vi "Sub_time_correction_2022.vi"(2 "Experimental Results IN":T1={"time_average_cycle"=0.0, "measured_frequency"=[], "date_time"="", "estimated_pin_node"=[], "time_cycle_start"=[], "measured_pin_location"=[], "estimated_frequency"=[], "acceleration_data"=[], "accelerometer_sample_rate"=0.0, "displacement_sample_rate"=0.0, "time_compare_start"=array[564 elements], "time_subsample_start"=array[564 elements], "time_FEA_start"=array[564 elements], "time_FEA_end"=array[564 elements], "time_cycle_end"=array[564 elements], "time_accelerometer_aquire_start"=array[564 elements], "time_frequency_calculations_start"=array[564 elements], "time_frequency_calculations_end"=array[564 elements], "measured_pin_location_tt"=array[564 elements], "time_ACC_data_collection_start"=0.0, "time_acceleration_data"=array[564 elements], "estimated_pin_location"=array[564 elements], "scaling_factor_Hz_per_pin_to_frequency_resolution"=1.0, "Std_Dev_equale_particles_divided_3"=TRUE, "Auto_FFT_length"=TRUE, "windowed_acc_data"=array1x564[564 elements], "FFT"=array1x564[564 elements]}) -> (16 "Experimental Results OUT":T1={"time_average_cycle"=0.0, "measured_frequency"=[], "date_time"="", "estimated_pin_node"=[], "time_cycle_start"=[], "measured_pin_location"=[], "estimated_frequency"=[], "acceleration_data"=[], "accelerometer_sample_rate"=0.0, "displacement_sample_rate"=0.0, "time_compare_start"=array[564 elements], "time_subsample_start"=array[564 elements], "time_FEA_start"=array[564 elements], "time_FEA_end"=array[564 elements], "time_cycle_end"=array[564 elements], "time_accelerometer_aquire_start"=array[564 elements], "time_frequency_calculations_start"=array[564 elements], "time_frequency_calculations_end"=array[564 elements], "measured_pin_location_tt"=array[564 elements], "time_ACC_data_collection_start"=0.0, "time_acceleration_data"=array[564 elements], "estimated_pin_location"=array[564 elements], "scaling_factor_Hz_per_pin_to_frequency_resolution"=1.0, "Std_Dev_equale_particles_divided_3"=TRUE, "Auto_FFT_length"=TRUE, "windowed_acc_data"=array1x564[564 elements], "FFT"=array1x564[564 elements]})   [LabVIEW 2019]
uses:
  <vilib>/Analysis/baseanly.llb/Mean (DBL).vi
  <vilib>/Analysis/NI_AALBase.lvlib
panel:
  out "mean":dbl format="%0.10f"
  out "number of iterations run":i32
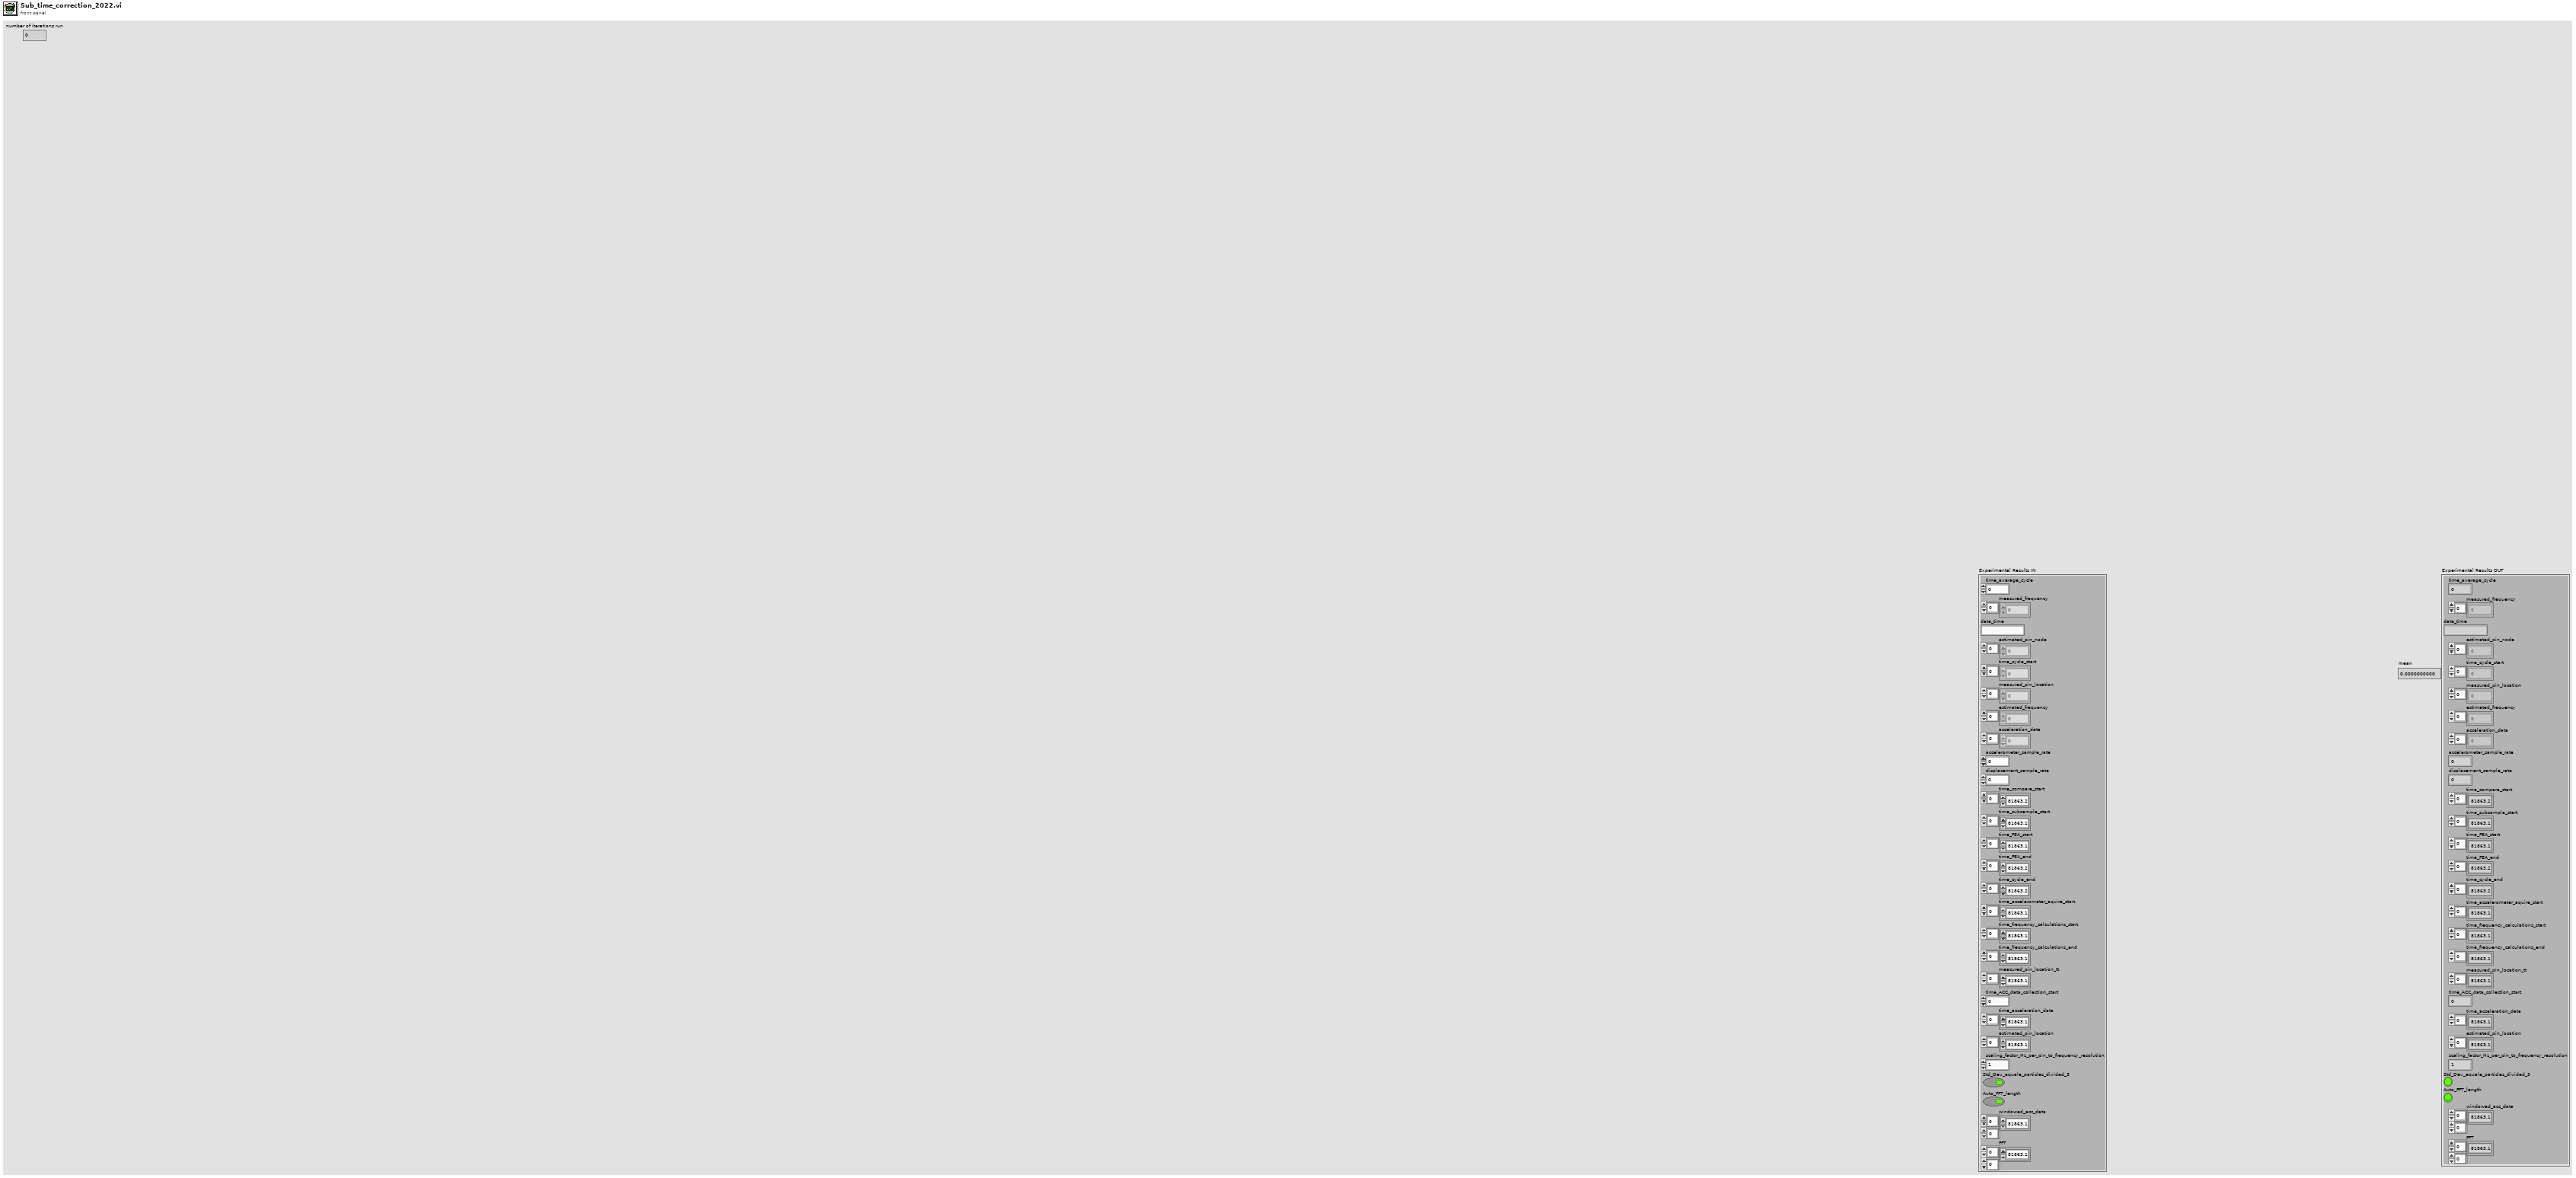
[diagram p1: front panel]
types:
  T1 = cluster{"time_average_cycle":dbl, "measured_frequency":dbl[], "date_time":string, "estimated_pin_node":i32[], "time_cycle_start":dbl[], "measured_pin_location":dbl[], "estimated_frequency":dbl[], "acceleration_data":dbl[], "accelerometer_sample_rate":dbl, "displacement_sample_rate":dbl, "time_compare_start":dbl[], "time_subsample_start":dbl[], "time_FEA_start":dbl[], "time_FEA_end":dbl[], "time_cycle_end":dbl[], "time_accelerometer_aquire_start":dbl[], "time_frequency_calculations_start":dbl[], "time_frequency_calculations_end":dbl[], "measured_pin_location_tt":dbl[], "time_ACC_data_collection_start":dbl, "time_acceleration_data":dbl[], "estimated_pin_location":dbl[], "scaling_factor_Hz_per_pin_to_frequency_resolution":dbl, "Std_Dev_equale_particles_divided_3":bool, "Auto_FFT_length":bool, "windowed_acc_data":dbl[][], "FFT":dbl[][]}
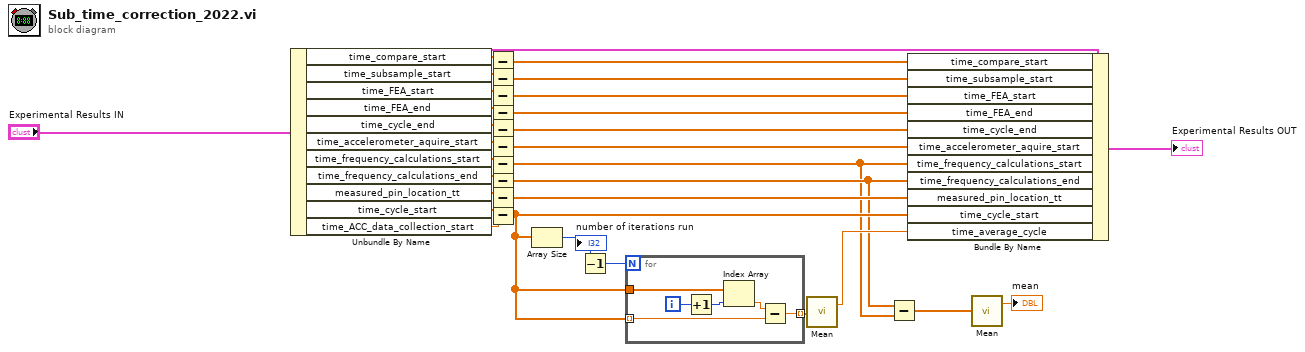
[diagram p0: block diagram]
diagram:
  n1 = Unbundle By Name("Experimental Results IN") -> ("time_compare_start"=w2:dbl[], "time_subsample_start"=w3:dbl[], "time_FEA_start"=w4:dbl[], "time_FEA_end"=w5:dbl[], "time_cycle_end"=w6:dbl[], "time_accelerometer_aquire_start"=w7:dbl[], "time_frequency_calculations_start"=w8:dbl[], "time_frequency_calculations_end"=w9:dbl[], "measured_pin_location_tt"=w10:dbl[], "time_cycle_start"=w11:dbl[], "time_ACC_data_collection_start"=w1:dbl)
  n2 = Subtract(x=w2, y=w1) -> (x-y=w29:dbl[])
  n3 = Subtract(x=w3, y=w1) -> (x-y=w28:dbl[])
  n4 = Subtract(x=w4, y=w1) -> (x-y=w27:dbl[])
  n5 = Subtract(x=w5, y=w1) -> (x-y=w23:dbl[])
  n6 = Subtract(x=w6, y=w1) -> (x-y=w26:dbl[])
  n7 = Subtract(x=w7, y=w1) -> (x-y=w25:dbl[])
  n8 = Subtract(x=w8, y=w1) -> (x-y=w16:dbl[])
  n9 = Subtract(x=w9, y=w1) -> (x-y=w17:dbl[])
  n10 = Subtract(x=w10, y=w1) -> (x-y=w24:dbl[])
  n11 = Subtract(x=w11, y=w1) -> (x-y=w18:dbl[])
  n12 = Array Size(array=w18) -> (size(s)=w21:i32)
  "number of iterations run" <- w21
  n13 = Decrement(x=w21) -> (x-1=w22:i32)
  n14 = for {
    N: w22 -> [_]
    tunnel: w18 -> [w35] mode=indexing
    tunnel: w18 -> [w34]
    tunnel: [w30] -> w20 mode=indexing
    i -> [w33]
    n15 = Increment(x=w33) -> (x+1=w32:i32)
    n16 = Index Array(array=w34, index=w32) -> (element=w31:dbl)
    n17 = Subtract(x=w31, y=w35) -> (x-y=w30:dbl)
  }
  n18 = call-poly <vilib>:"Mean.vi"("X"=w20) -> ("mean"=w19:dbl)  [unwired: 1 out]
  n19 = Subtract(x=w17, y=w16) -> (x-y=w15:dbl[])
  n20 = Bundle By Name(cluster="Experimental Results IN", "time_compare_start"=w29, "time_subsample_start"=w28, "time_FEA_start"=w27, "time_FEA_end"=w23, "time_cycle_end"=w26, "time_accelerometer_aquire_start"=w25, "time_frequency_calculations_start"=w16, "time_frequency_calculations_end"=w17, "measured_pin_location_tt"=w24, "time_cycle_start"=w18, "time_average_cycle"=w19) -> (→"Experimental Results OUT":T1)
  n21 = call-poly <vilib>:"Mean.vi"("X"=w15) -> ("mean"=→"mean":dbl)  [unwired: 1 out]
